vi "Read Representation.vi"(9 "Numeric in":refnum<class "Numeric.lvclass">) -> (3 "Numeric out":refnum<class "Numeric.lvclass">, 4 "Numeric Representation":T1)   [LabVIEW 2014, in "Raspberry Pi Compatible Compiler for LabVIEW.lvlib" / "Numeric.lvclass"]
uses:
  Numeric.lvclass
  <vilib>/numeric/LVNumericRepresentation.ctl
  Numeric.lvclass/Numeric.ctl
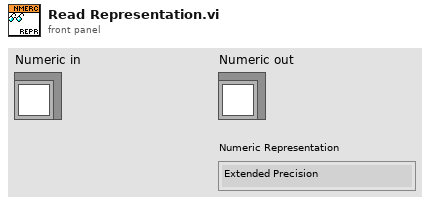
[diagram p1: front panel]
types:
  T1 = typedef "LVNumericRepresentation.ctl" = enum32{"Extended Precision", "Double Precision", "Single Precision", "Long", "Word", "Byte", "Unsigned Long", "Unsigned Word", "Unsigned Byte", "Complex Extended", "Complex Double", "Complex Single", "Quad", "Unsigned Quad", "Fixed-Point"}
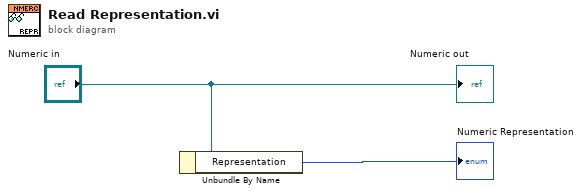
[diagram p0: block diagram]
diagram:
  n1 = Unbundle By Name("Numeric in") -> ("Representation"=→"Numeric Representation":T1)
  "Numeric out" <- "Numeric in"
